vi "Destroy.vi"(8 "Error In":errorcluster, 11 "reference in":refnum<class "Customer.lvclass">) -> (0 "Error Out":errorcluster, 3 "reference out":refnum<class "Customer.lvclass">)   [LabVIEW 2020, in "Customer.lvclass"]
uses:
  Customer.lvclass
  Colleague_class/Colleague.lvclass
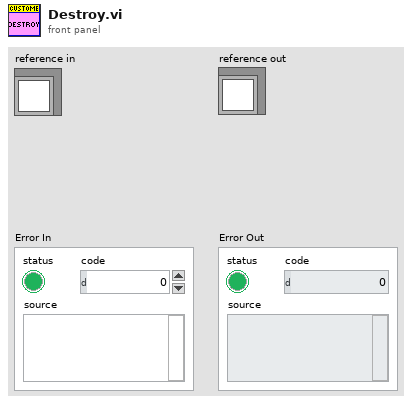
[diagram p1: front panel]
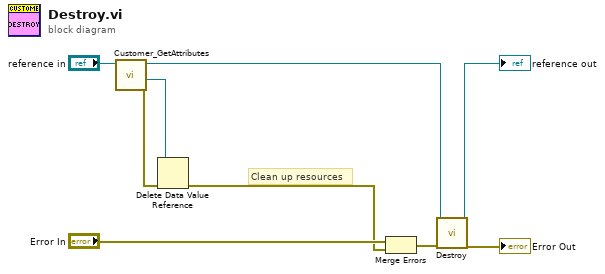
[diagram p0: block diagram]
diagram:
  # "Clean up resources"
  n1 = call "Customer_GetAttributes.vi"("reference in"="reference in") -> ("error out"=w7:errorcluster, "DataRef"=w5:refnum<data-value>, "reference out"=w6:refnum<class "Customer.lvclass">)  [unwired: 7 in, 1 out]
  n2 = Delete Data Value Reference(data value reference=w5, error in=w7) -> (error out=w3:errorcluster)  [unwired: 1 out]
  n3 = Merge Errors("Error In", w3) -> (w9:errorcluster)
  n4 = call-parent "Destroy.vi"("Error In"=w9, "reference in"=w6) -> ("Error Out"=→"Error Out":errorcluster, "reference out"=→"reference out":refnum<class "Customer.lvclass">)  [unwired: 8 in]
